vi "ILABs_CaseHandlerNoPath.vi"(2 "error In":errorcluster, 3 "appReference":refnum<vi>, 4 "data":string, 5 "action":string) -> (0 "errorOut":string, 1 "response":string)   [LabVIEW 2009]
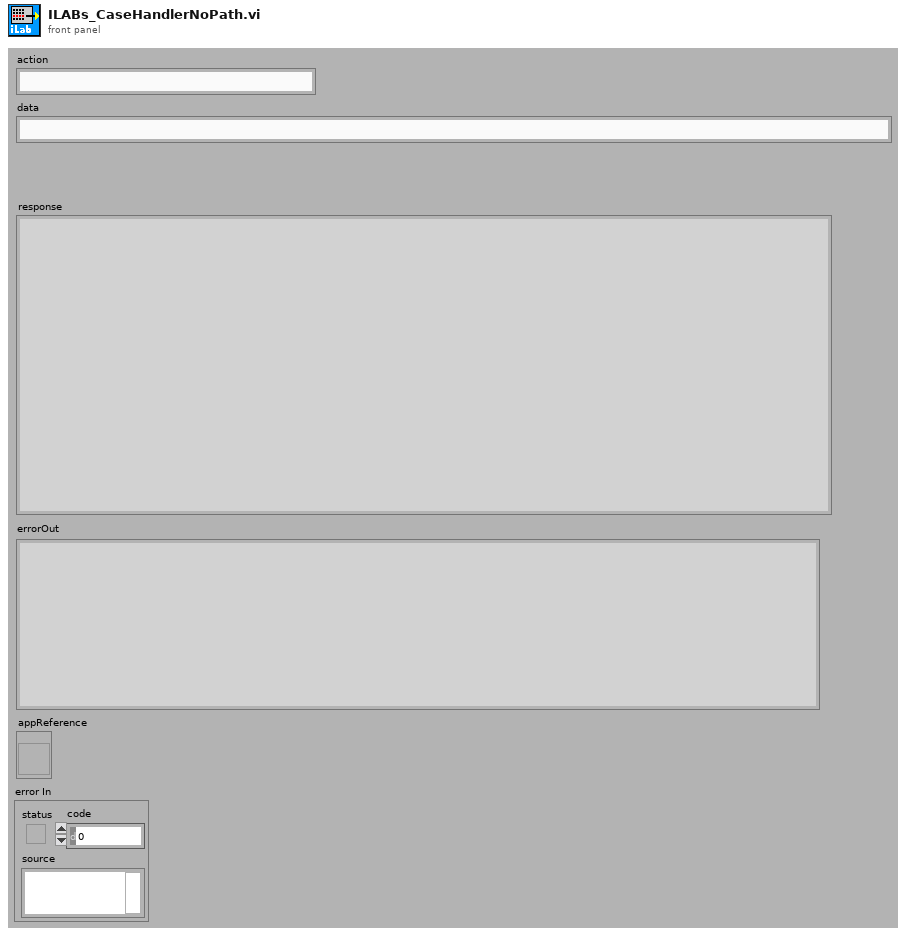
[diagram p1: front panel]
types:
  T1 = enum32{"Bad", "Idle", "Run top level", "Running"}
  T2 = typedef "LVRemotePanelConnectionsTypeDef.ctl" = cluster{"VI Name":string, "Remote":string, "UserName":string, "Port":i32, "Status":enum32{"Viewing", "Waiting For Control", "Controlling"}, "Create Time":timestamp, "Status Time":timestamp, "Control End Time":timestamp}[]
  T3 = cluster{"VI Name":string, "Remote":string, "UserName":string, "Port":i32, "Status":enum32{"Viewing", "Waiting For Control", "Controlling"}, "Create Time":timestamp, "Status Time":timestamp, "Control End Time":timestamp}
  T4 = cluster{"Name":string, "Path":path, "Type String":string, "Display Name":string, "Type":string}
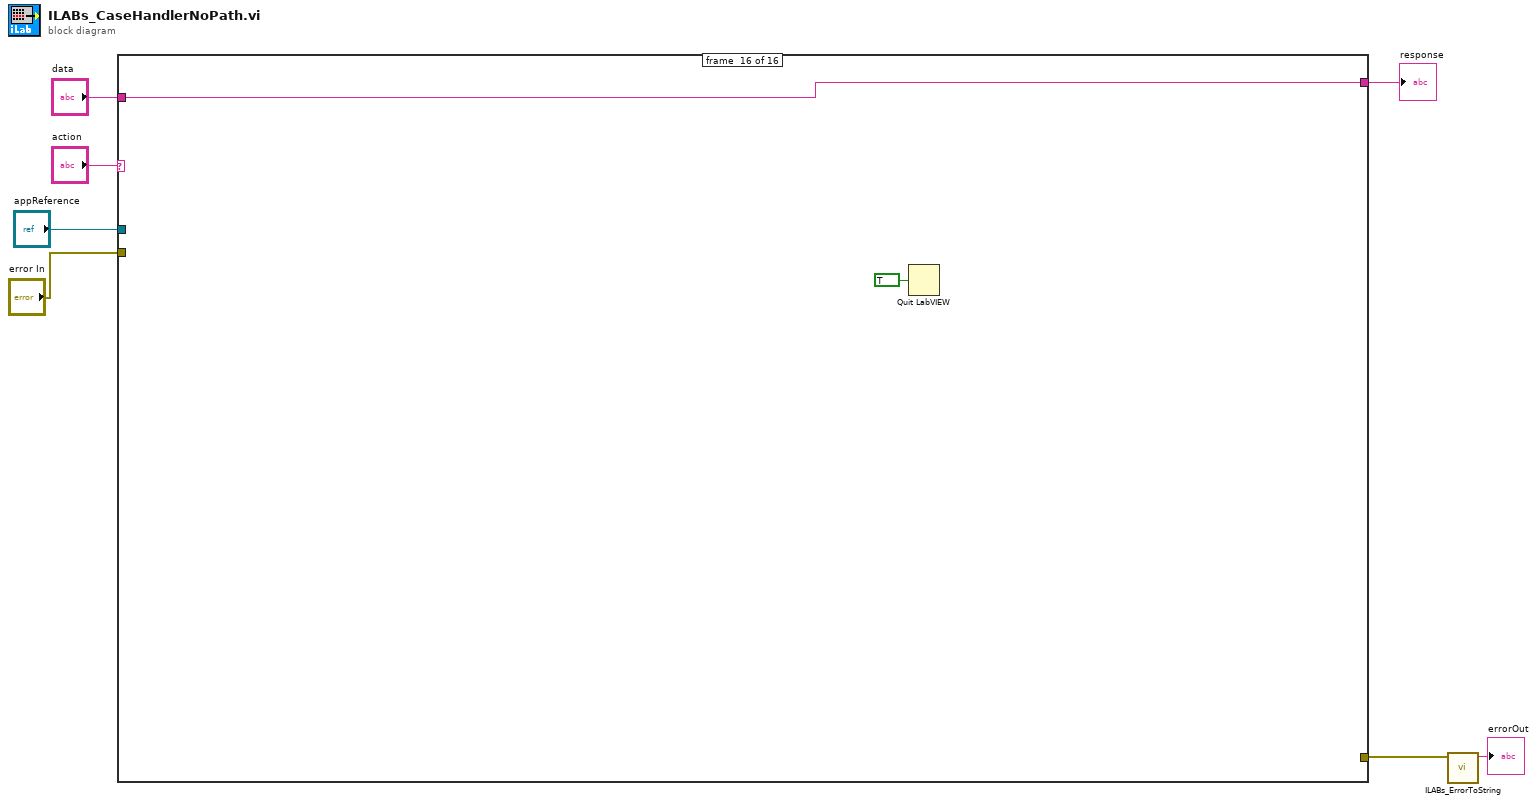
[diagram p0: block diagram]
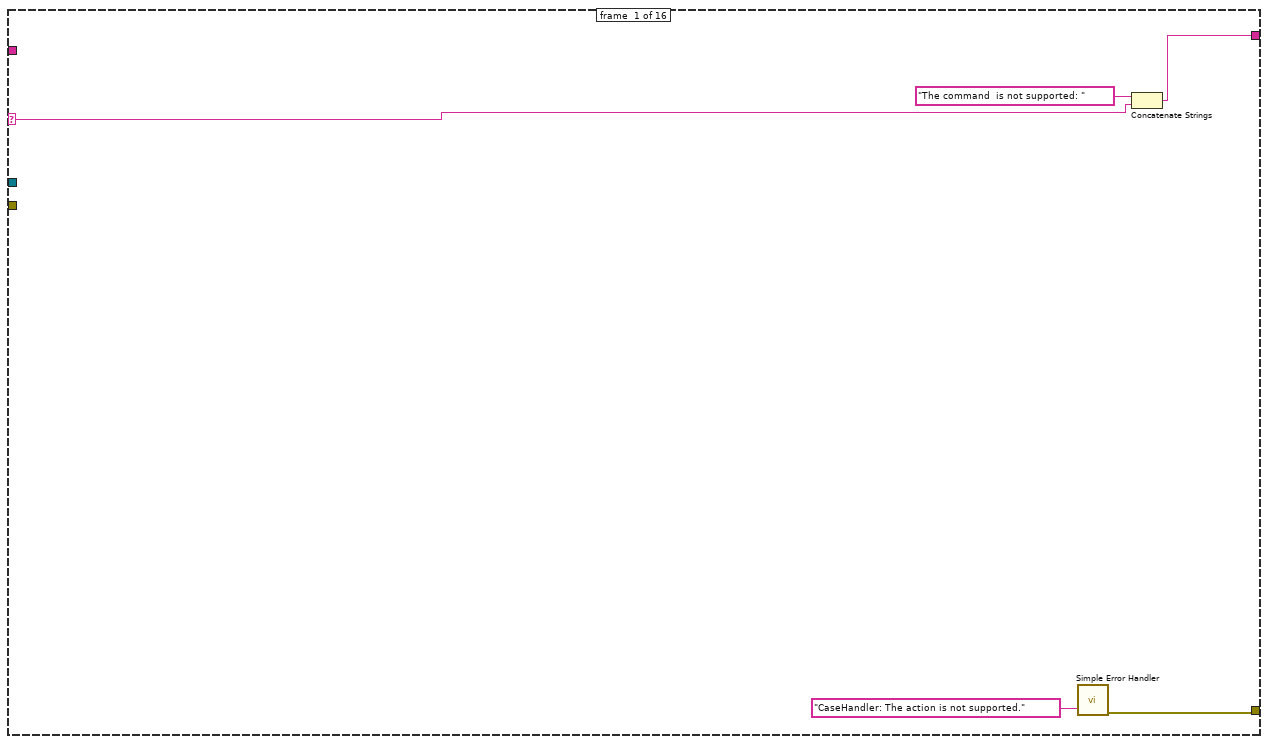
[diagram p2: hidden frame]
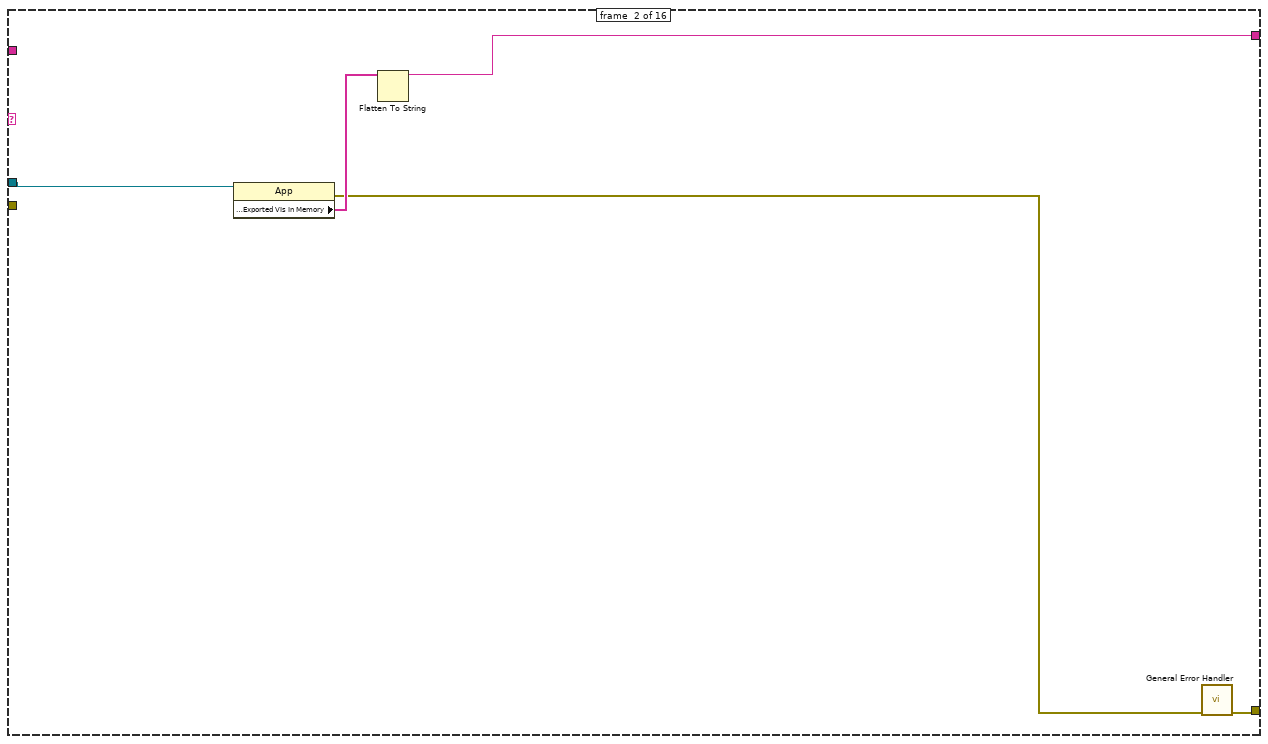
[diagram p3: hidden frame]
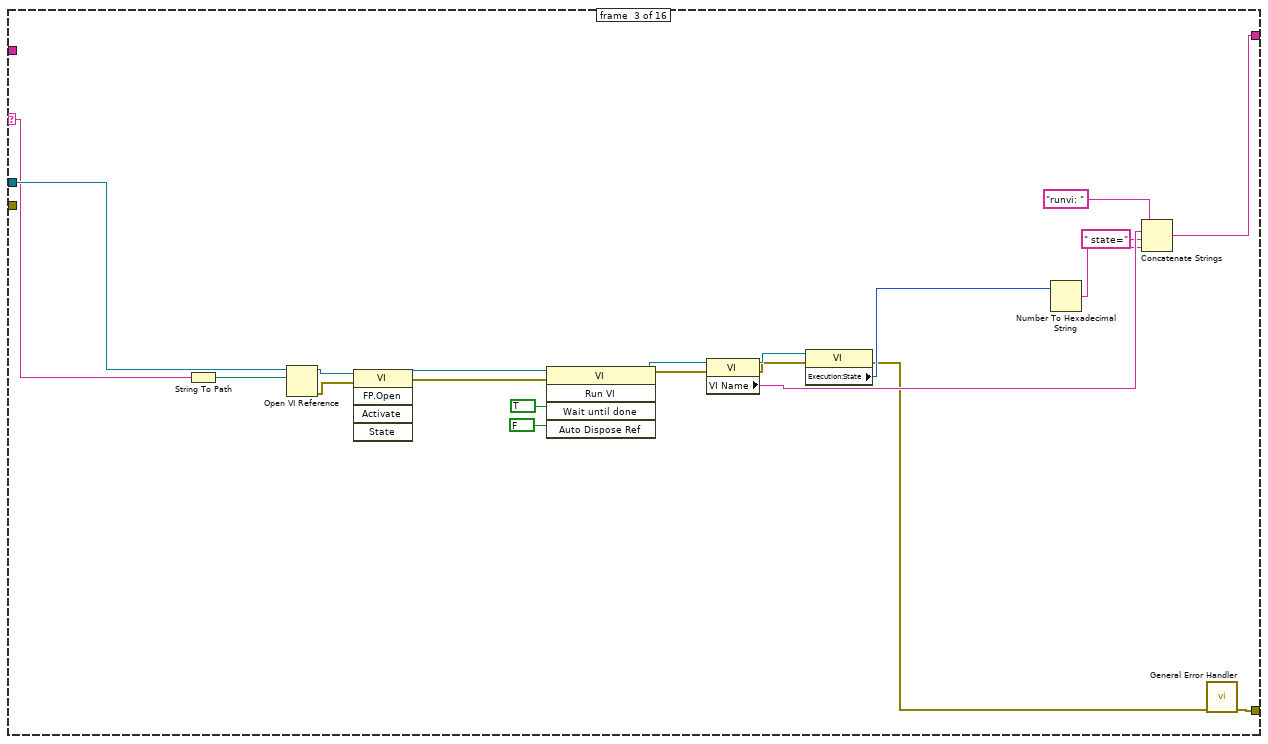
[diagram p4: hidden frame]
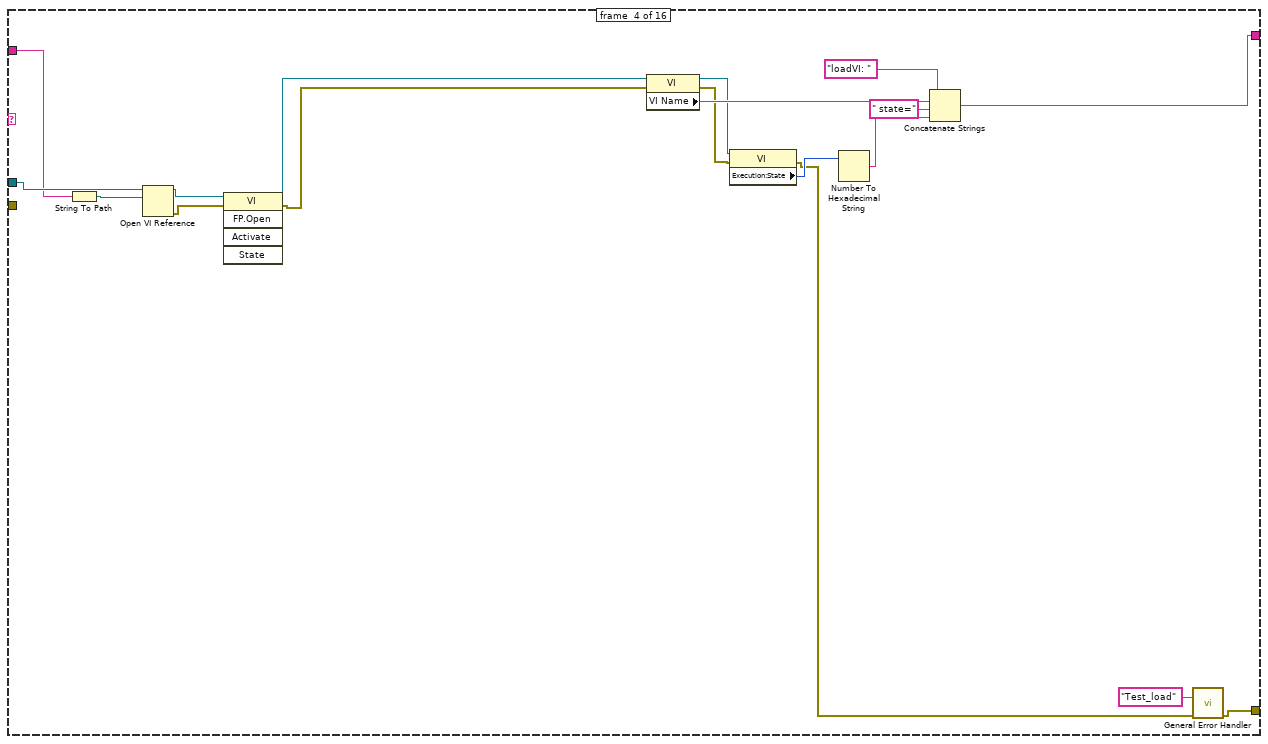
[diagram p5: hidden frame]
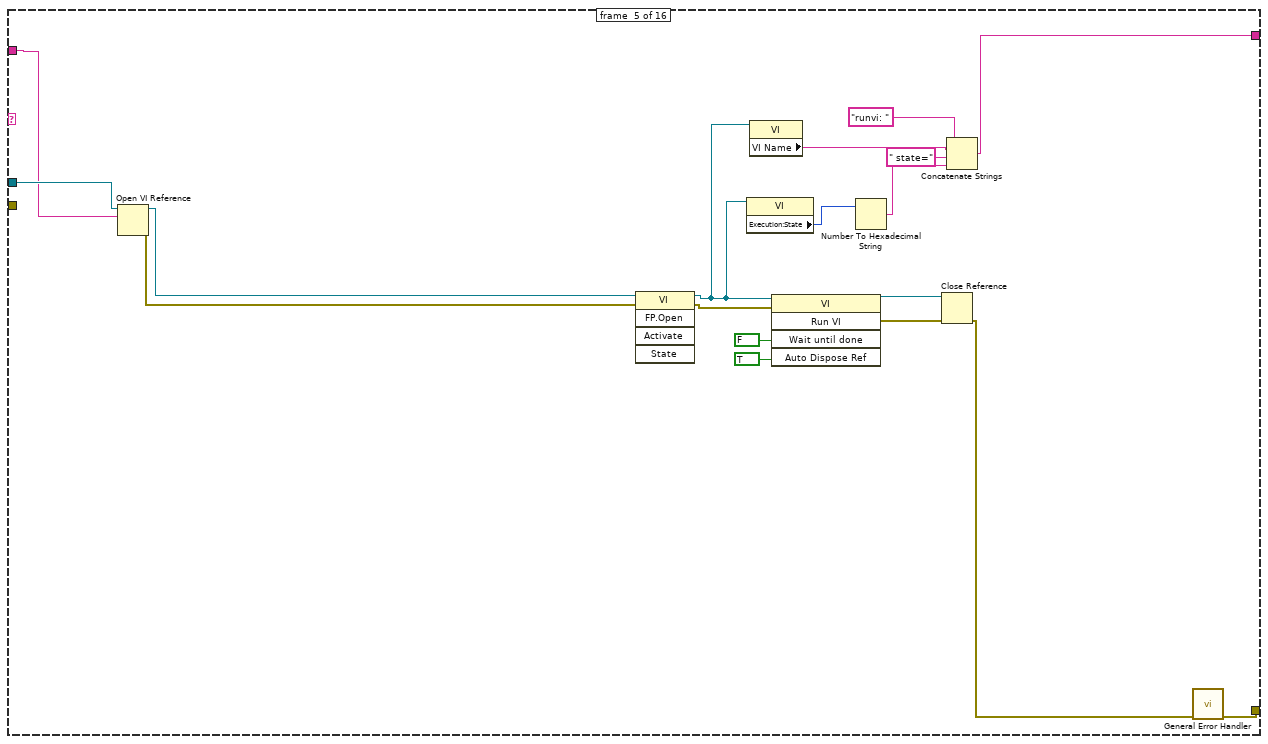
[diagram p6: hidden frame]
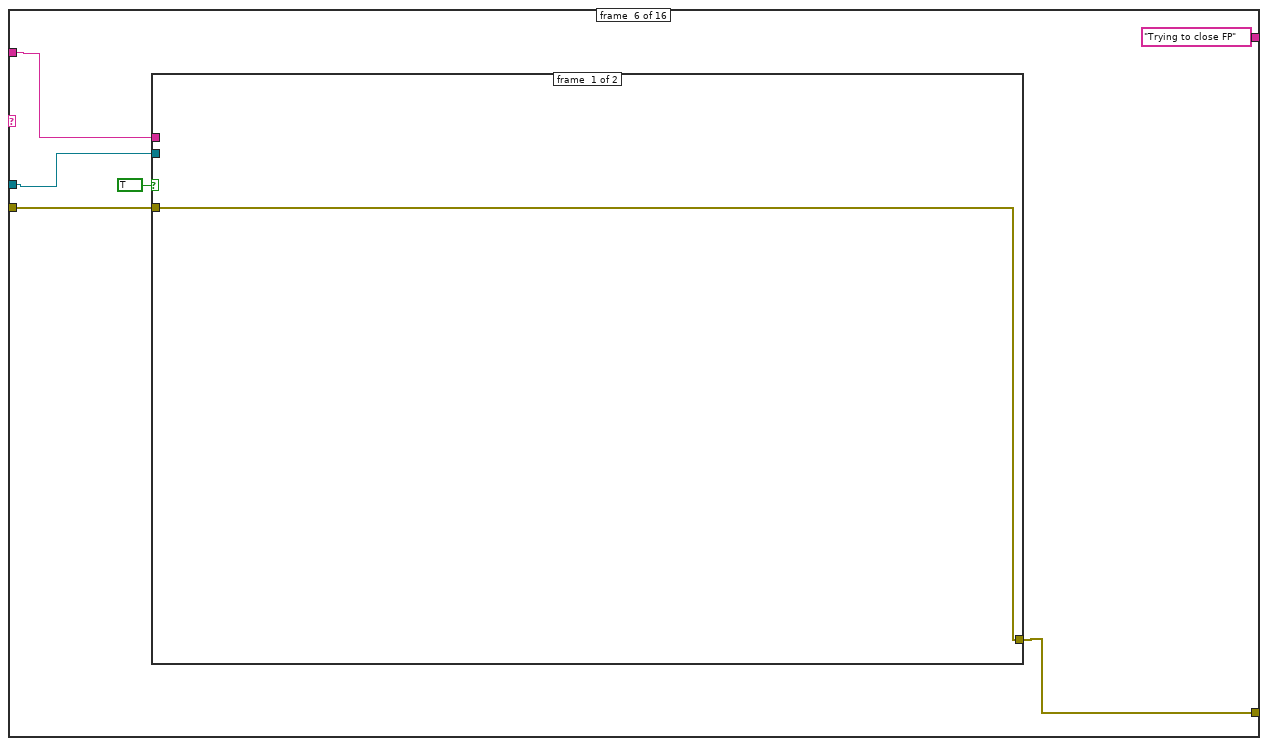
[diagram p7: hidden frame]
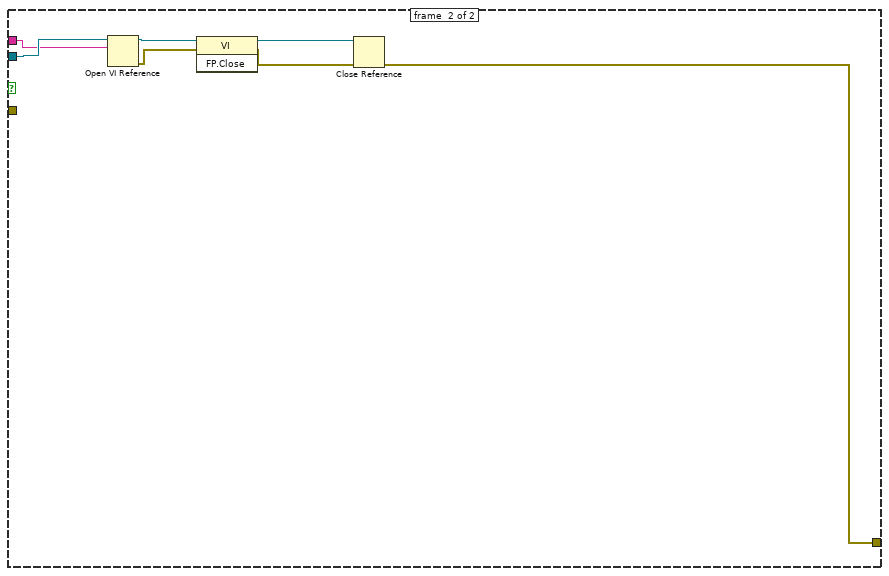
[diagram p8: hidden frame]
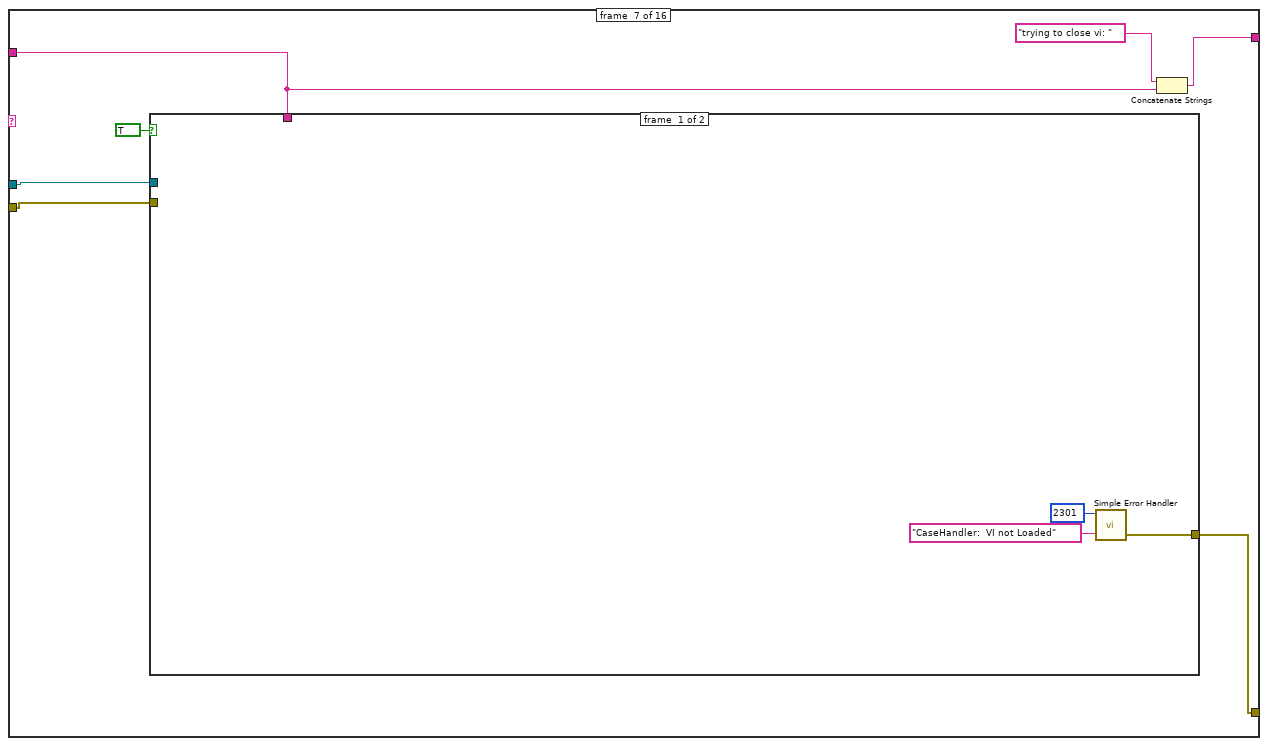
[diagram p9: hidden frame]
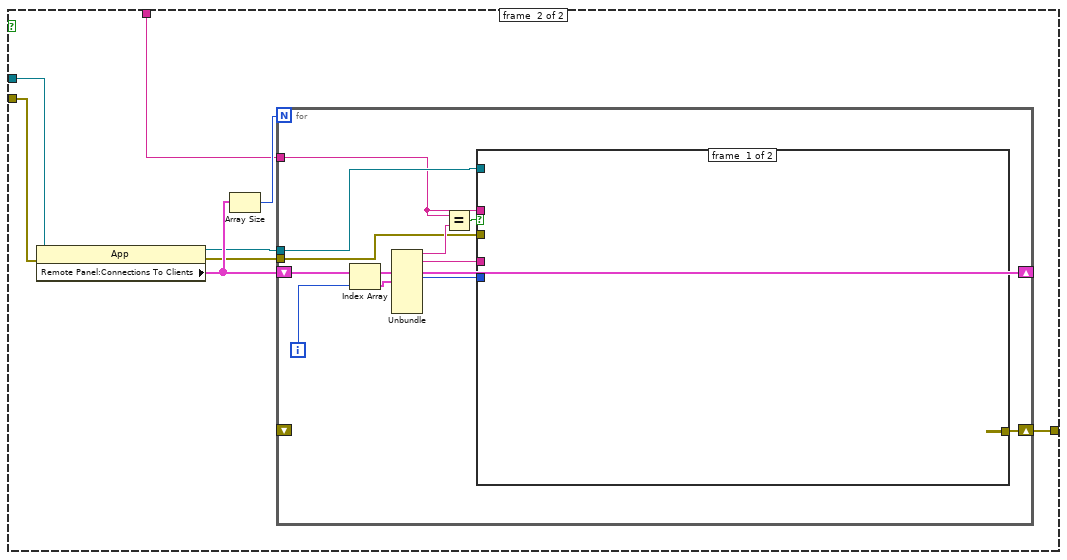
[diagram p10: hidden frame]
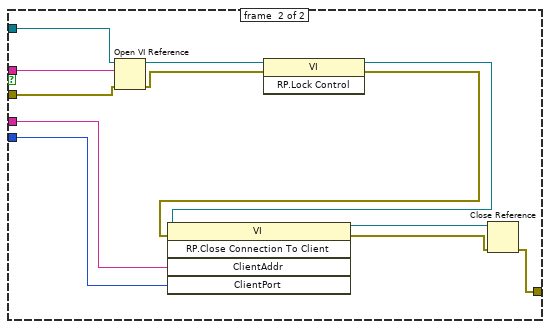
[diagram p11: hidden frame]
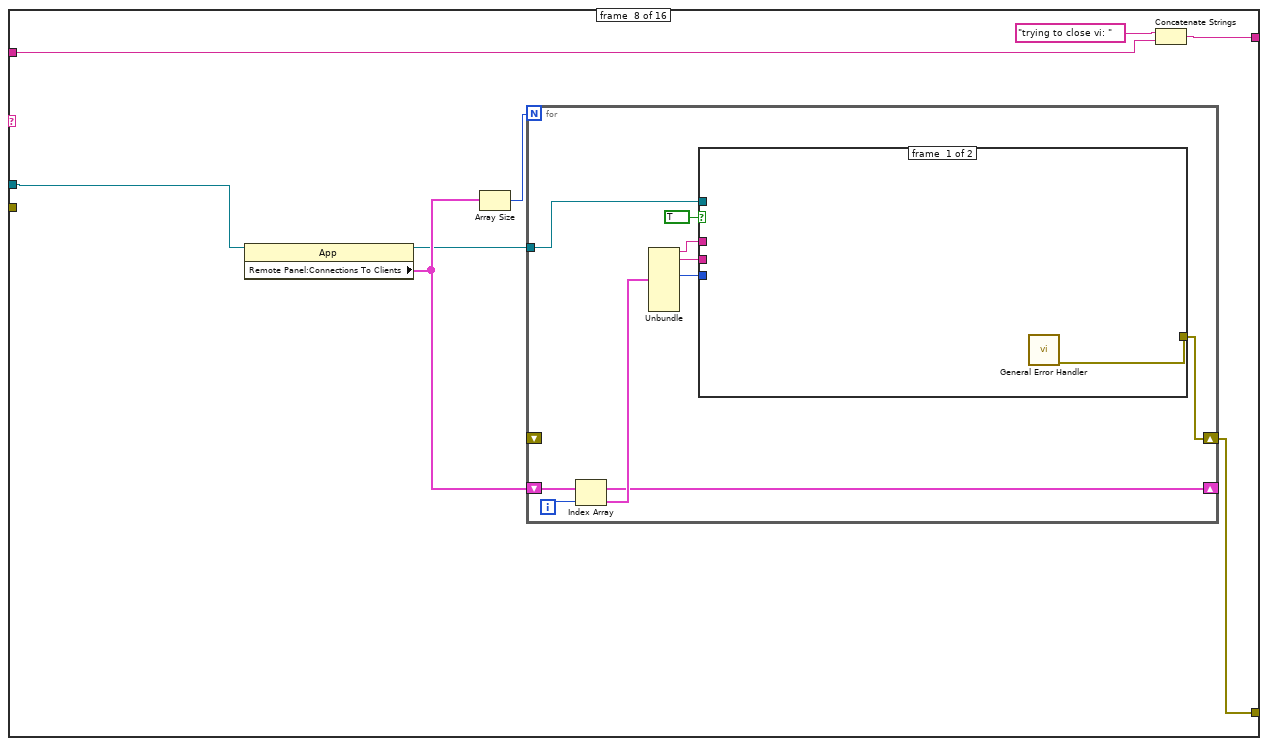
[diagram p12: hidden frame]
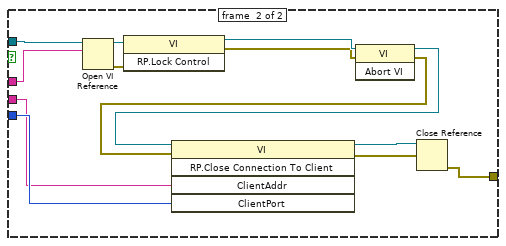
[diagram p13: hidden frame]
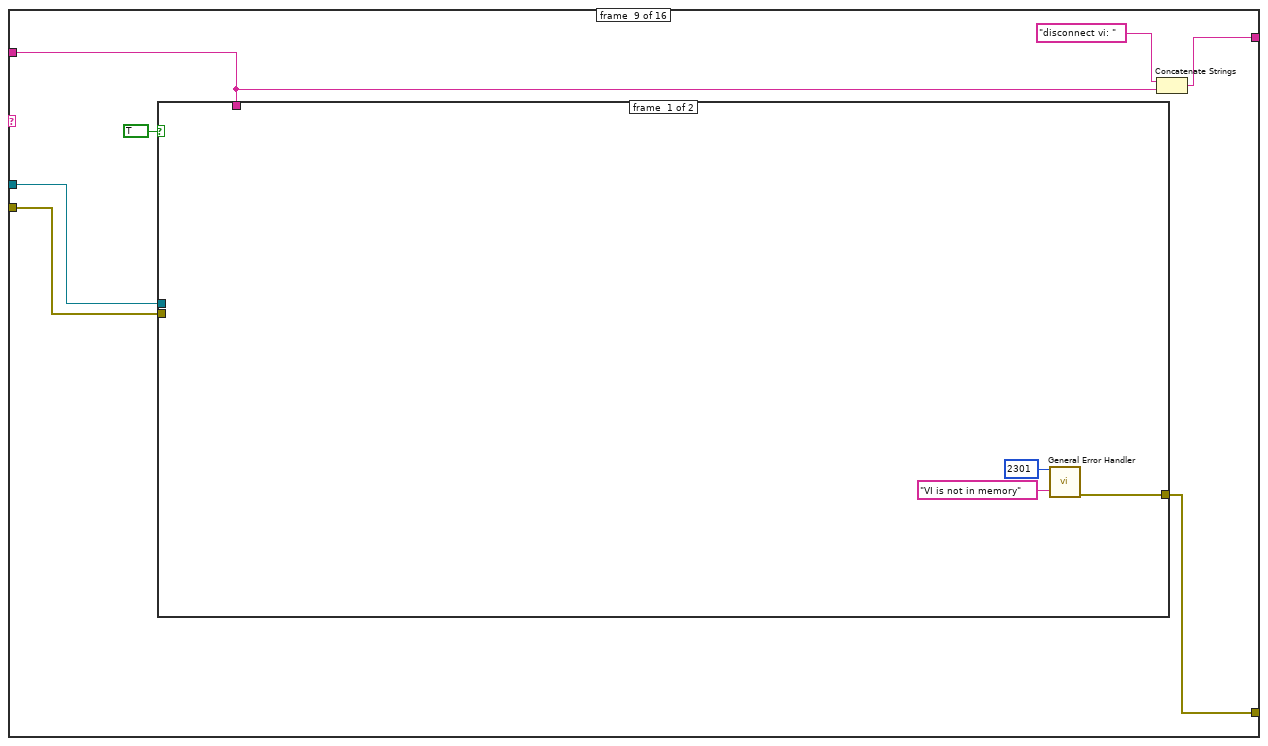
[diagram p14: hidden frame]
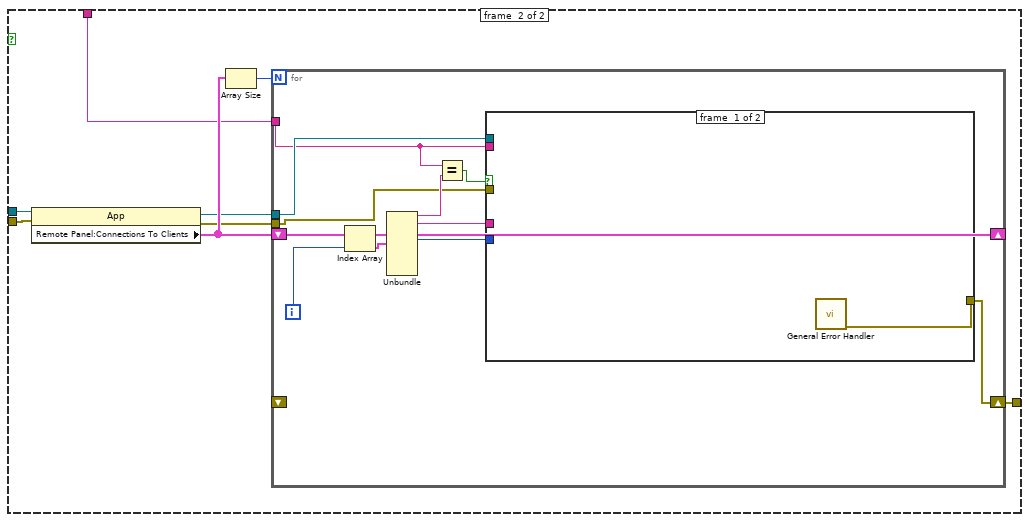
[diagram p15: hidden frame]
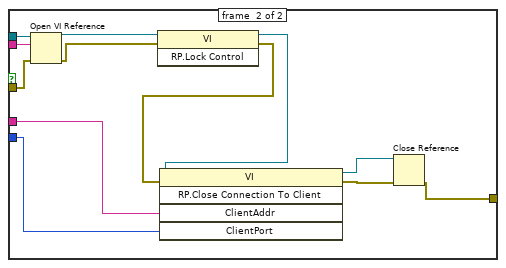
[diagram p16: hidden frame]
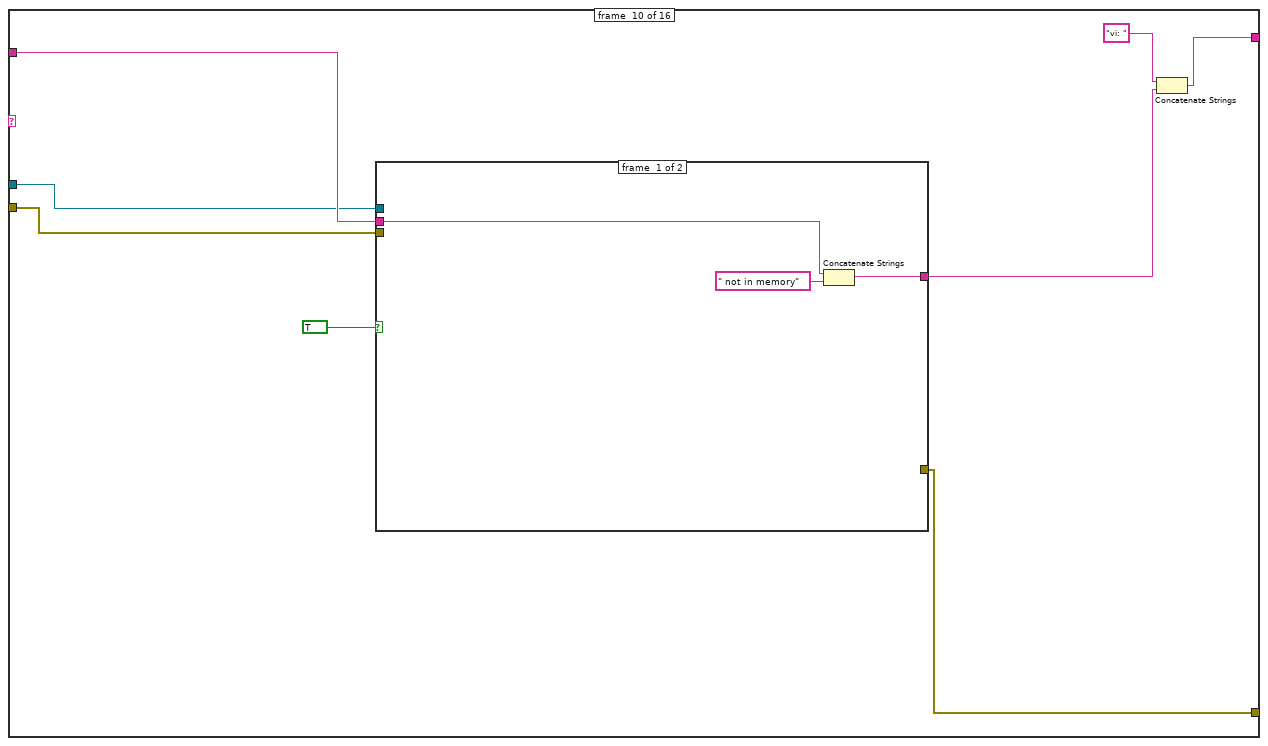
[diagram p17: hidden frame]
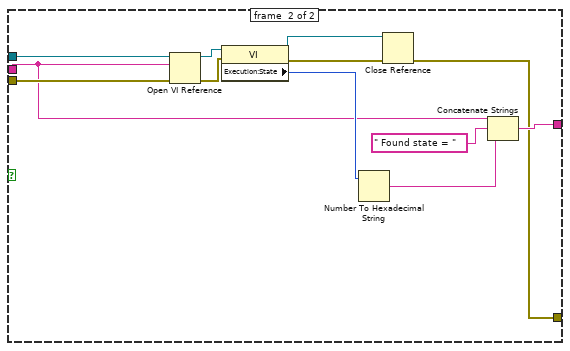
[diagram p18: hidden frame]
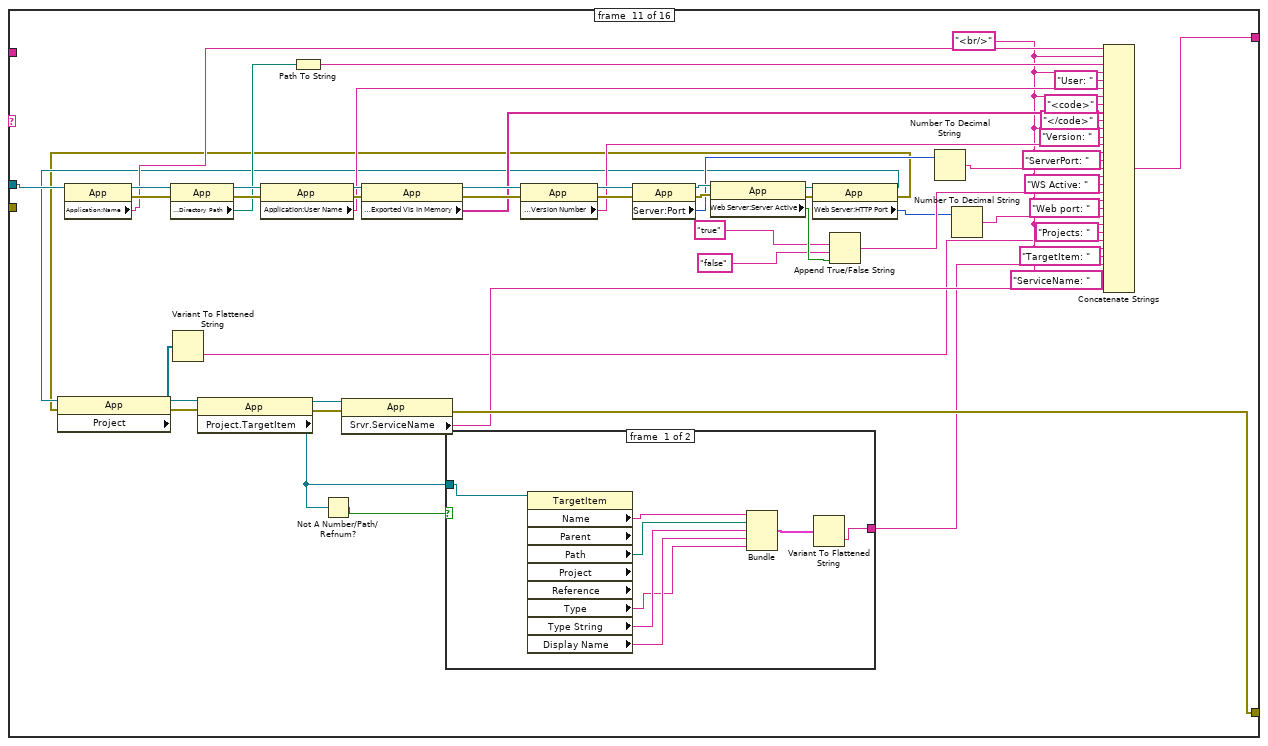
[diagram p19: hidden frame]
diagram:
  n1 = case shown="\"appstatus\"" "action" {
    selector: "action" -> [w11 _ w18 _ _ _ _ _ _ _ _ _ _ _ _ _]
    tunnel: "data" -> [_ _ _ w39 w57 w80 w92 w134 w164 w207 _ w288 w300 w318 w332 w355]
    tunnel: [w10 w17 w30 w50 w65 "Trying to close FP" ("data") w94 w133 w166 w210 w243 w299 w317 w328 w336 w355] -> w6
    tunnel: [w8 w14 w28 w49 w62 w78 w93 w132 w165 w206 w236 w290 w309 w319 w333 _] -> w4
    tunnel: "appReference" -> [_ w13 w27 w48 w61 w79 w91 w131 w163 w205 w279 w289 w305 w320 w331 _]
    tunnel: "error In" -> [_ _ _ _ _ w75 w90 _ w161 w204 _ w292 w306 _ w330 _]
    frame #0 {
      (unwired) "The" ("message")
      n2 = call <vilib>:"Simple Error Handler.vi"("error source (\" \")"="CaseHandler: The action is not supported." ("error source (\" \")")) -> ("error out"=w8:errorcluster)  [unwired: 2 in, 6 out]
      n3 = Concatenate Strings("The command  is not supported: " ("string"), w11) -> (w10:string)
    }
    frame #1 {
      n4 = property class="App"(reference=w13) -> (error out=w15:errorcluster, "Application:Exported VIs In Memory"=w16:string[])  [unwired: 1 in, 1 out]
      n5 = Flatten To String(anything=w16) -> (data string=w17:string)  [unwired: 1 in, 4 out]
      n6 = call <vilib>:"General Error Handler.vi"("error in (no error)"=w15) -> ("error out"=w14:errorcluster)  [unwired: 1 in, 13 out]
    }
    frame #2 {
      n7 = String To Path(string=w18) -> (path=w19:path)
      n8 = Open VI Reference(application reference (local)=w27, vi path=w19) -> (vi reference=w37:refnum<vi>, error out=w36:errorcluster)  [unwired: 1 in, 3 out]
      n9 = invoke class="VI" method="FP.Open"(reference=w37, error in=w36) -> (reference out=w26:refnum<vi>, error out=w25:errorcluster)  [unwired: 3 in, 3 out]
      n10 = invoke class="VI" method="Run VI"(reference=w26, error in=w25, "Wait until done"=FALSE, "Auto Dispose Ref"=TRUE) -> (reference out=w24:refnum<vi>, error out=w23:errorcluster)  [unwired: 1 in, 3 out]
      n11 = property class="VI"(reference=w24, error in=w23) -> (reference out=w22:refnum<vi>, error out=w21:errorcluster, "VI Name"=w35:string)
      n12 = property class="VI"(reference=w22, error in=w21) -> (error out=w20:errorcluster, "Execution:State"=w33:T1)  [unwired: 1 out]
      n13 = Number To Hexadecimal String(2:w33) -> (0:w32:string)  [unwired: 1 out]
      n14 = Concatenate Strings("runvi: " ("string"), w35, " state=" ("string"), w32) -> (w30:string)
      n15 = call <vilib>:"General Error Handler.vi"("error in (no error)"=w20) -> ("error out"=w28:errorcluster)  [unwired: 1 in, 13 out]
    }
    frame #3 {
      n16 = String To Path(string=w39) -> (path=w40:path)
      n17 = Open VI Reference(application reference (local)=w48, vi path=w40) -> (vi reference=w44:refnum<vi>, error out=w43:errorcluster)  [unwired: 1 in, 3 out]
      n18 = invoke class="VI" method="FP.Open"(reference=w44, error in=w43) -> (reference out=w42:refnum<vi>, error out=w41:errorcluster)  [unwired: 3 in, 3 out]
      n19 = property class="VI"(reference=w42, error in=w41) -> (reference out=w46:refnum<vi>, error out=w47:errorcluster, "VI Name"=w55:string)
      n20 = property class="VI"(reference=w46, error in=w47) -> (error out=w45:errorcluster, "Execution:State"=w53:T1)  [unwired: 1 out]
      n21 = Number To Hexadecimal String(2:w53) -> (0:w52:string)  [unwired: 1 out]
      n22 = Concatenate Strings("loadVI: " ("string"), w55, " state=" ("string"), w52) -> (w50:string)
      n23 = call <vilib>:"General Error Handler.vi"("[error source] (\" \")"="Test_load" ("[error source] (\" \")"), "error in (no error)"=w45) -> ("error out"=w49:errorcluster)  [unwired: 1 in, 12 out]
    }
    frame #4 {
      w63 = TRUE items=["OFF", "ON", "OFF", "ON"] ("Auto Dispose Ref")
      n24 = Open VI Reference(application reference (local)=w61, vi path=w57) -> (vi reference=w73:refnum<vi>, error out=w71:errorcluster)  [unwired: 1 in, 3 out]
      n25 = invoke class="VI" method="FP.Open"(reference=w73, error in=w71) -> (reference out=w70:refnum<vi>, error out=w72:errorcluster)  [unwired: 3 in, 3 out]
      n26 = property class="VI"(reference=w70) -> ("Execution:State"=w67:T1)  [unwired: 1 in, 2 out]
      n27 = property class="VI"(reference=w70) -> ("VI Name"=w69:string)  [unwired: 1 in, 2 out]
      n28 = invoke class="VI" method="Run VI"(reference=w70, error in=w72, "Wait until done"=FALSE, "Auto Dispose Ref"=w63) -> (reference out=w58:refnum<vi>, error out=w59:errorcluster)  [unwired: 1 in, 3 out]
      n29 = Number To Hexadecimal String(2:w67) -> (0:w66:string)  [unwired: 1 out]
      n30 = Close Reference(reference=w58, error in (no error)=w59) -> (error out=w60:errorcluster)
      n31 = Concatenate Strings("runvi: " ("string"), w69, " state=" ("string"), w66) -> (w65:string)
      n32 = call <vilib>:"General Error Handler.vi"("error in (no error)"=w60) -> ("error out"=w62:errorcluster)  [unwired: 1 in, 13 out]
    }
    frame #5 {
      n33 = case shown="True" TRUE {
        tunnel: w80 -> [_ w82]
        tunnel: w79 -> [_ w88]
        tunnel: [w81 w83] -> w78
        tunnel: w75 -> [w81 _]
        frame #0 {
        }
        frame #1 {
          n34 = Open VI Reference(application reference (local)=w88, vi path=w82) -> (vi reference=w87:refnum<vi>, error out=w86:errorcluster)  [unwired: 1 in, 3 out]
          n35 = invoke class="VI" method="FP.Close"(reference=w87, error in=w86) -> (reference out=w85:refnum<vi>, error out=w84:errorcluster)  [unwired: 1 in, 1 out]
          n36 = Close Reference(reference=w85, error in (no error)=w84) -> (error out=w83:errorcluster)
        }
      }
    }
    frame #6 {
      n37 = case shown="True" TRUE {
        tunnel: [w98 w104] -> w93
        tunnel: w92 -> [_ w103]
        tunnel: w90 -> [_ w101]
        tunnel: w91 -> [_ w102]
        frame #0 {
          n38 = call <vilib>:"Simple Error Handler.vi"("error code (no error:0)"=2301, "error source (\" \")"="CaseHandler:  VI not Loaded" ("error source (\" \")")) -> ("error out"=w98:errorcluster)  [unwired: 2 in, 5 out]
        }
        frame #1 {
          n39 = property class="App"(reference=w102, error in=w101) -> (reference out=w100:refnum<vi>, error out=w99:errorcluster, "Remote Panel:Connections To Clients"=w105:T2)
          n40 = Array Size(array=w105) -> (size(s)=w106:i32)
          n41 = for {
            N: w106 -> [_]
            shift-right: [w110] -> _
            shift-left: w105 -> [w110]
            tunnel: w103 -> [w108]
            shift-right: [w112] -> w104
            shift-left: _ -> [_]
            tunnel: w100 -> [w109]
            tunnel: w99 -> [w107]
            i -> [w117]
            n42 = Index Array(array=w110, index=w117) -> (element=w116:T3)
            n43 = Unbundle(w116) -> ("VI Name"=w111:string, "Remote"=w113:string, "Port"=w114:i32)  [unwired: 5 out]
            n44 = Equal?(x=w108, y=w111) -> (x = y?=w115:bool)
            n45 = case shown="True" w115 {
              tunnel: w114 -> [_ w129]
              tunnel: w113 -> [_ w128]
              tunnel: [_ w127] -> w112
              tunnel: w109 -> [_ w124]
              tunnel: w108 -> [_ w123]
              tunnel: w107 -> [_ w120]
              frame #0 {
              }
              frame #1 {
                n46 = Open VI Reference(application reference (local)=w124, vi path=w123, error in (no error)=w120) -> (vi reference=w119:refnum<vi>, error out=w118:errorcluster)  [unwired: 3 out]
                n47 = invoke class="VI" method="RP.Lock Control"(reference=w119, error in=w118) -> (reference out=w122:refnum<vi>, error out=w121:errorcluster)  [unwired: 1 in, 1 out]
                n48 = invoke class="VI" method="RP.Close Connection To Client"(reference=w122, error in=w121, "ClientAddr"=w128, "ClientPort"=w129) -> (reference out=w125:refnum<vi>, error out=w126:errorcluster)  [unwired: 1 in, 3 out]
                n49 = Close Reference(reference=w125, error in (no error)=w126) -> (error out=w127:errorcluster)
              }
            }
          }
        }
      }
      n50 = Concatenate Strings("trying to close vi: " ("data"), w92) -> (w94:string)
    }
    frame #7 {
      n51 = property class="App"(reference=w131) -> (reference out=w130:refnum<vi>, "Remote Panel:Connections To Clients"=w136:T2)  [unwired: 1 in, 1 out]
      n52 = Array Size(array=w136) -> (size(s)=w137:i32)
      n53 = for {
        N: w137 -> [_]
        shift-right: [w140] -> _
        shift-left: w136 -> [w140]
        shift-right: [w142] -> w132
        shift-left: _ -> [_]
        tunnel: w130 -> [w139]
        i -> [w146]
        n54 = Index Array(array=w140, index=w146) -> (element=w145:T3)
        n55 = Unbundle(w145) -> ("VI Name"=w141:string, "Remote"=w143:string, "Port"=w144:i32)  [unwired: 5 out]
        n56 = case shown="True" TRUE {
          tunnel: w144 -> [_ w160]
          tunnel: w143 -> [_ w159]
          tunnel: [w147 w158] -> w142
          tunnel: w141 -> [_ w157]
          tunnel: w139 -> [_ w148]
          frame #0 {
            n57 = call <vilib>:"General Error Handler.vi"() -> ("error out"=w147:errorcluster)  [unwired: 2 in, 13 out]
          }
          frame #1 {
            n58 = Open VI Reference(application reference (local)=w148, vi path=w157) -> (vi reference=w152:refnum<vi>, error out=w151:errorcluster)  [unwired: 1 in, 3 out]
            n59 = invoke class="VI" method="RP.Lock Control"(reference=w152, error in=w151) -> (reference out=w150:refnum<vi>, error out=w149:errorcluster)  [unwired: 1 in, 1 out]
            n60 = invoke class="VI" method="Abort VI"(reference=w150, error in=w149) -> (reference out=w153:refnum<vi>, error out=w154:errorcluster)  [unwired: 1 in, 1 out]
            n61 = invoke class="VI" method="RP.Close Connection To Client"(reference=w153, error in=w154, "ClientAddr"=w159, "ClientPort"=w160) -> (reference out=w156:refnum<vi>, error out=w155:errorcluster)  [unwired: 1 in, 3 out]
            n62 = Close Reference(reference=w156, error in (no error)=w155) -> (error out=w158:errorcluster)
          }
        }
      }
      n63 = Concatenate Strings("trying to close vi: " ("data"), w134) -> (w133:string)
    }
    frame #8 {
      n64 = case shown="True" TRUE {
        tunnel: [w170 w176] -> w165
        tunnel: w164 -> [_ w175]
        tunnel: w163 -> [_ w174]
        tunnel: w161 -> [_ w172]
        frame #0 {
          n65 = call <vilib>:"General Error Handler.vi"("[error code] (0)"=2301, "[error source] (\" \")"="VI is not in memory" ("[error source] (\" \")")) -> ("error out"=w170:errorcluster)  [unwired: 2 in, 11 out]
        }
        frame #1 {
          n66 = property class="App"(reference=w174, error in=w172) -> (reference out=w173:refnum<vi>, error out=w171:errorcluster, "Remote Panel:Connections To Clients"=w177:T2)
          n67 = Array Size(array=w177) -> (size(s)=w178:i32)
          n68 = for {
            N: w178 -> [_]
            shift-right: [w182] -> _
            shift-left: w177 -> [w182]
            tunnel: w175 -> [w179]
            shift-right: [w184] -> w176
            shift-left: _ -> [_]
            tunnel: w173 -> [w181]
            tunnel: w171 -> [w180]
            i -> [w189]
            n69 = Index Array(array=w182, index=w189) -> (element=w188:T3)
            n70 = Unbundle(w188) -> ("VI Name"=w183:string, "Remote"=w185:string, "Port"=w186:i32)  [unwired: 5 out]
            n71 = Equal?(x=w179, y=w183) -> (x = y?=w187:bool)
            n72 = case shown="True" w187 {
              tunnel: w186 -> [_ w202]
              tunnel: w185 -> [_ w201]
              tunnel: [w190 w193] -> w184
              tunnel: w181 -> [_ w196]
              tunnel: w180 -> [_ w192]
              tunnel: w179 -> [_ w191]
              frame #0 {
                n73 = call <vilib>:"General Error Handler.vi"() -> ("error out"=w190:errorcluster)  [unwired: 2 in, 13 out]
              }
              frame #1 {
                n74 = Open VI Reference(application reference (local)=w196, vi path=w191, error in (no error)=w192) -> (vi reference=w200:refnum<vi>, error out=w197:errorcluster)  [unwired: 3 out]
                n75 = invoke class="VI" method="RP.Lock Control"(reference=w200, error in=w197) -> (reference out=w199:refnum<vi>, error out=w198:errorcluster)  [unwired: 1 in, 1 out]
                n76 = invoke class="VI" method="RP.Close Connection To Client"(reference=w199, error in=w198, "ClientAddr"=w201, "ClientPort"=w202) -> (reference out=w194:refnum<vi>, error out=w195:errorcluster)  [unwired: 1 in, 3 out]
                n77 = Close Reference(reference=w194, error in (no error)=w195) -> (error out=w193:errorcluster)
              }
            }
          }
        }
      }
      n78 = Concatenate Strings("disconnect vi: " ("data"), w164) -> (w166:string)
    }
    frame #9 {
      n79 = case shown="True" TRUE {
        tunnel: w207 -> [w213 w214]
        tunnel: [_ w216] -> w206
        tunnel: [w212 w221] -> w208
        tunnel: w205 -> [_ w219]
        tunnel: w204 -> [_ w215]
        frame #0 {
          n80 = Concatenate Strings(w213, " not in memory" ("string")) -> (w212:string)
        }
        frame #1 {
          n81 = Open VI Reference(application reference (local)=w219, vi path=w214, error in (no error)=w215) -> (vi reference=w225:refnum<vi>, error out=w224:errorcluster)  [unwired: 3 out]
          n82 = property class="VI"(reference=w225, error in=w224) -> (reference out=w218:refnum<vi>, error out=w217:errorcluster, "Execution:State"=w223:T1)
          n83 = Number To Hexadecimal String(2:w223) -> (0:w222:string)  [unwired: 1 out]
          n84 = Close Reference(reference=w218, error in (no error)=w217) -> (error out=w216:errorcluster)
          n85 = Concatenate Strings(w214, " Found state = " ("string"), w222) -> (w221:string)
        }
      }
      n86 = Concatenate Strings("vi: " ("data"), w208) -> (w210:string)
    }
    frame #10 {
      w234 = "<br/>" ("string")
      n87 = property class="App"(reference=w279) -> (reference out=w278:refnum<vi>, error out=w273:errorcluster, "Application:Name"=w264:string)  [unwired: 1 in]
      n88 = property class="App"(reference=w278, error in=w273) -> (reference out=w277:refnum<vi>, error out=w272:errorcluster, "Application:Directory Path"=w262:path)
      n89 = property class="App"(reference=w277, error in=w272) -> (reference out=w276:refnum<vi>, error out=w271:errorcluster, "Application:User Name"=w260:string)
      n90 = Path To String(path=w262) -> (string=w263:string)
      n91 = property class="App"(reference=w276, error in=w271) -> (reference out=w275:refnum<vi>, error out=w270:errorcluster, "Application:Exported VIs In Memory"=w258:string[])
      n92 = property class="App"(reference=w275, error in=w270) -> (reference out=w274:refnum<vi>, error out=w269:errorcluster, "Application:Version Number"=w255:string)
      n93 = property class="App"(reference=w274, error in=w269) -> (reference out=w265:refnum<vi>, error out=w266:errorcluster, "Server:Port"=w252:u32)
      n94 = property class="App"(reference=w265, error in=w266) -> (reference out=w268:refnum<vi>, error out=w267:errorcluster, "Web Server:Server Active"=w250:bool)
      n95 = property class="App"(reference=w268, error in=w267) -> (reference out=w242:refnum<vi>, error out=w239:errorcluster, "Web Server:HTTP Port"=w245:u16)
      n96 = property class="App"(reference=w242, error in=w239) -> (reference out=w241:refnum<vi>, error out=w238:errorcluster, "Project"=w230:refnum<vi>[])
      n97 = Variant To Flattened String(Variant=w230) -> (data string=w229:string)  [unwired: 1 out]
      n98 = property class="App"(reference=w241, error in=w238) -> (reference out=w240:refnum<vi>, error out=w237:errorcluster, "Project.TargetItem"=w226:refnum<vi>)
      n99 = Not A Number/Path/Refnum?(number/path/refnum=w226) -> (NaN/Path/Refnum?=w227:bool)
      n100 = property class="App"(reference=w240, error in=w237) -> (error out=w236:errorcluster, "Srvr.ServiceName"=w231:string)  [unwired: 1 out]
      n101 = case shown="True" w227 {
        tunnel: [w281 _] -> w228
        tunnel: w226 -> [w280 _]
        frame #0 {
          n102 = property class="TargetItem" props=["Name", "Parent", "Path", "Project", "Reference", "Type", "Type String", "Display Name"](reference=w280) -> ("Name"=w287:string, "Path"=w286:path, "Type"=w283:string, "Type String"=w285:string, "Display Name"=w284:string)  [unwired: 1 in, 5 out]
          n103 = Bundle("Name"=w287, "Path"=w286, "Type String"=w285, "Display Name"=w284, "Type"=w283) -> (w282:T4)  [unwired: 1 out]
          n104 = Variant To Flattened String(Variant=w282) -> (data string=w281:string)  [unwired: 1 out]
        }
        frame #1 {
        }
      }
      n105 = Append True/False String(1:w250, 2:"false" ("false string"), 3:"true" ("true string")) -> (0:w249:string)  [unwired: 1 out]
      n106 = Number To Decimal String(number=w252) -> (decimal integer string=w253:string)  [unwired: 1 out]
      n107 = Number To Decimal String(number=w245) -> (decimal integer string=w244:string)  [unwired: 1 out]
      n108 = Concatenate Strings(w264, w234, w263, w234, "User: " ("string"), w260, w234, "<code>" ("string"), w258, "</code>" ("string"), w234, "Version: " ("string"), w255, w234, "ServerPort: " ("string"), w253, w234, "WS Active: " ("string"), w249, w234, "Web port: " ("string"), w244, w234, "Projects: " ("string"), w229, w234, "TargetItem: " ("string"), w228, w234, "ServiceName: " ("string"), w231) -> (w243:string)
    }
    frame #11 {
      n109 = Open VI Reference(application reference (local)=w289, vi path=w288, error in (no error)=w292) -> (vi reference=w297:refnum<vi>, error out=w296:errorcluster)  [unwired: 3 out]
      n110 = invoke class="VI" method="RP.Lock Control"(reference=w297, error in=w296) -> (reference out=w294:refnum<vi>, error out=w293:errorcluster)  [unwired: 1 in, 1 out]
      n111 = Close Reference(reference=w294, error in (no error)=w293) -> (error out=w290:errorcluster)
      n112 = Concatenate Strings(w288, ": lock Control requested " ("string")) -> (w291:string)
      n113 = Concatenate Strings("vi: " ("data"), w291) -> (w299:string)
    }
    frame #12 {
      n114 = property class="App"(reference=w305, error in=w306) -> (reference out=w304:refnum<vi>, error out=w301:errorcluster, "WebSrvr.Port"=w308:u16)
      n115 = invoke class="App" method="RP.Client Release Control"(reference=w304, error in=w301, "VIName"=w300, "ServerAddress"="thrush.mit.edu" ("Server Address"), "ServerPort"=w308) -> (reference out=w302:refnum<vi>, error out=w303:errorcluster)  [unwired: 1 in, 4 out]
      n116 = Open VI Reference(application reference (local)=w302, vi path=w300, error in (no error)=w303) -> (vi reference=w315:refnum<vi>, error out=w314:errorcluster)  [unwired: 3 out]
      n117 = invoke class="VI" method="RP.Lock Control"(reference=w315, error in=w314) -> (reference out=w312:refnum<vi>, error out=w311:errorcluster)  [unwired: 1 in, 1 out]
      n118 = Close Reference(reference=w312, error in (no error)=w311) -> (error out=w309:errorcluster)
      n119 = Concatenate Strings(w300, ": lock Control requested " ("string")) -> (w310:string)
      n120 = Concatenate Strings("vi: " ("data"), w310) -> (w317:string)
    }
    frame #13 {
      n121 = Open VI Reference(application reference (local)=w320, vi path=w318) -> (vi reference=w326:refnum<vi>, error out=w325:errorcluster)  [unwired: 1 in, 3 out]
      n122 = invoke class="VI" method="RP.Unlock Control"(reference=w326, error in=w325) -> (reference out=w323:refnum<vi>, error out=w322:errorcluster)  [unwired: 1 in, 1 out]
      n123 = Concatenate Strings(w318, ": unlock requested " ("string")) -> (w321:string)
      n124 = Close Reference(reference=w323, error in (no error)=w322) -> (error out=w319:errorcluster)
      n125 = Concatenate Strings("vi: " ("data"), w321) -> (w328:string)
    }
    frame #14 {
      n126 = case shown="True" TRUE {
        tunnel: w332 -> [w339 w340]
        tunnel: [_ w344] -> w333
        tunnel: [w338 w351] -> w334
        tunnel: w331 -> [_ w347]
        tunnel: w330 -> [_ w341]
        frame #0 {
          n127 = Concatenate Strings(w339, " not in memory" ("string")) -> (w338:string)
        }
        frame #1 {
          n128 = Open VI Reference(application reference (local)=w347, vi path=w340, error in (no error)=w341) -> (vi reference=w343:refnum<vi>, error out=w342:errorcluster)  [unwired: 1 in, 2 out]
          n129 = invoke class="VI" method="Abort VI"(reference=w343, error in=w342) -> (reference out=w349:refnum<vi>, error out=w348:errorcluster)  [unwired: 1 in, 1 out]
          n130 = property class="VI"(reference=w349, error in=w348) -> (reference out=w346:refnum<vi>, error out=w345:errorcluster, "Execution:State"=w353:T1)
          n131 = Close Reference(reference=w346, error in (no error)=w345) -> (error out=w344:errorcluster)
          n132 = Number To Hexadecimal String(2:w353) -> (0:w352:string)  [unwired: 1 out]
          n133 = Concatenate Strings(w340, " Found state = " ("string"), w352) -> (w351:string)
        }
      }
      n134 = Concatenate Strings("stopvi: " ("data"), w334) -> (w336:string)
    }
    frame #15 {
      n135 = Quit LabVIEW(quit? (T)=TRUE) -> ()
    }
  }
  "response" <- w6
  n136 = call "ILABs_ErrorToString.vi"("errorIn"=w4) -> ("errorOut"=→"errorOut":string)  [unwired: 10 out]
